vi "PH_gentec_Powermeter.evt call Set Zero.vi"(0 "i ref in":refnum<vi>, 2 "Instance":string, 5 "error in (no error)":errorcluster) -> (14 "i ref out":refnum<vi>, 19 "error out":errorcluster)   [LabVIEW 2014, in "PH_gentec_Powermeter.lvlib"]
doc: "This VI sets the display to zero by a simple call."
uses:
  PH_gentec_Powermeter.lvlib
  CSCore/BaseProcess/BaseProcess.lvlib
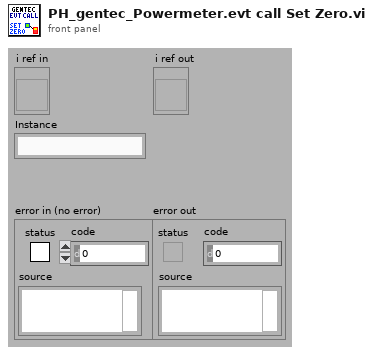
[diagram p1: front panel]
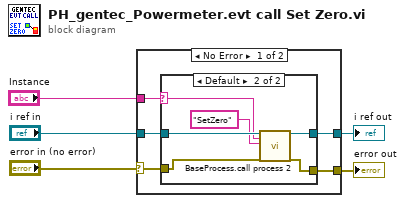
[diagram p0: block diagram]
diagram:
  n1 = case shown="No Error" "error in (no error)" {
    selector: "error in (no error)" -> [w6 w19]
    tunnel: [w10 w20] -> w1
    tunnel: [w9 w19] -> w2
    tunnel: "i ref in" -> [w8 w20]
    tunnel: "Instance" -> [w7 _]
    frame No Error {
      n2 = case shown="Default" w7 {
        selector: w7 -> [_ w13]
        tunnel: [w12 w18] -> w10
        tunnel: [w11 w17] -> w9
        tunnel: w8 -> [w12 w16]
        tunnel: w6 -> [w11 w15]
        frame "N/A" {
        }
        frame Default {
          n3 = call "BaseProcess.call process 2.vi"("i ref in"=w16, "Object"=w13, "Selector"="SetZero", "error in (no error)"=w15) -> ("i ref out"=w18:refnum<vi>, "error out"=w17:errorcluster)  [unwired: 14 in]
        }
      }
    }
    frame Error {
    }
  }
  "error out" <- w2
  "i ref out" <- w1
